vi "Configure Integer Display Dialog.vi"(7 "DisplayFilter":u8(ring)=7 items=["K_CHAN_R", "K_CHAN_W", "K_CHAN_RW", "K_CHAN_VOLT", "K_CHAN_FAULT", "K_ALL", "K_CUSTOM", "K_CHAN_R_VIS", "K_CHAN_W_VIS", "K_CHAN_RW_VIS", "K_CHAN_VOLT_VIS", "K_CHAN_FAULT_VIS"], 8 "error in (no error)":errorcluster, 9 "NIVS.System Definition Root":refnum<k24>, 11 "Data cluster in":T1={"Node Path"="", "NodePathArray"=[], "Integer"={"Label"="", "Digits of Precision"=0, "Integer Format"=enum."Scientific"}}) -> (0 "error out":errorcluster, 3 "Data cluster out":T1={"Node Path"="", "NodePathArray"=[], "Integer"={"Label"="", "Digits of Precision"=0, "Integer Format"=enum."Scientific"}})   [LabVIEW 2012]
doc: "Use this template to create a dialog box with event handling."
uses:
  NationalInstruments.VeriStand.SystemStorageUI
  NationalInstruments.VeriStand.SystemStorage
  <vilib>/NI Veristand/UI Controls/Single Node Browser/NI_VS UI Single Node Browser.lvlib
panel:
  in  "Integer Format":u8(ring) items=["Decimal"=0, "Scientific"=8, "Engineering"=2, "Binary"=3, "Octal"=4, "Hexadecimal"=5]
  in  "Digits of Precision":u8
  in  "Cancel":bool
  in  "Ok":bool
  in  "Selected Channel":refnum<k24>(container)
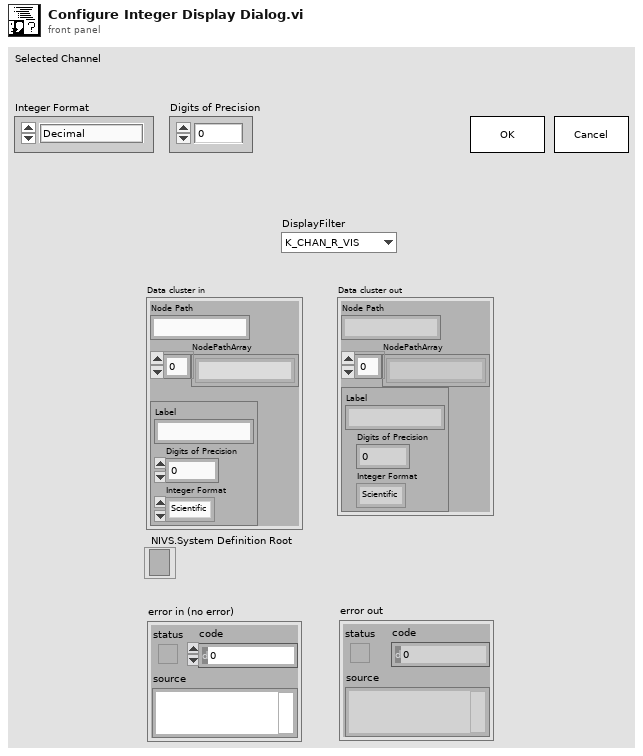
[diagram p1: front panel]
types:
  T1 = cluster{"Node Path":string, "NodePathArray":string[], "Integer":cluster{"Label":string, "Digits of Precision":u8, "Integer Format":enum8{"Decimal", "Scientific", "Engineering", "Binary", "Octal", "Hexadecimal", "Relative Time", "Time and Date", "SI"}}}
  T2 = enum8{"Decimal", "Scientific", "Engineering", "Binary", "Octal", "Hexadecimal", "Relative Time", "Time and Date", "SI"}
  T3 = typedef "NI_VS UI Single Node Browser.lvlib/Callback Type.ctl" = cluster{"Net Callbacks":refnum<k27>[], "Event":refnum<user-event>}
  T4 = typedef "NI_VS UI Single Node Browser.lvlib/Node Ref.ctl" = refnum<k24>
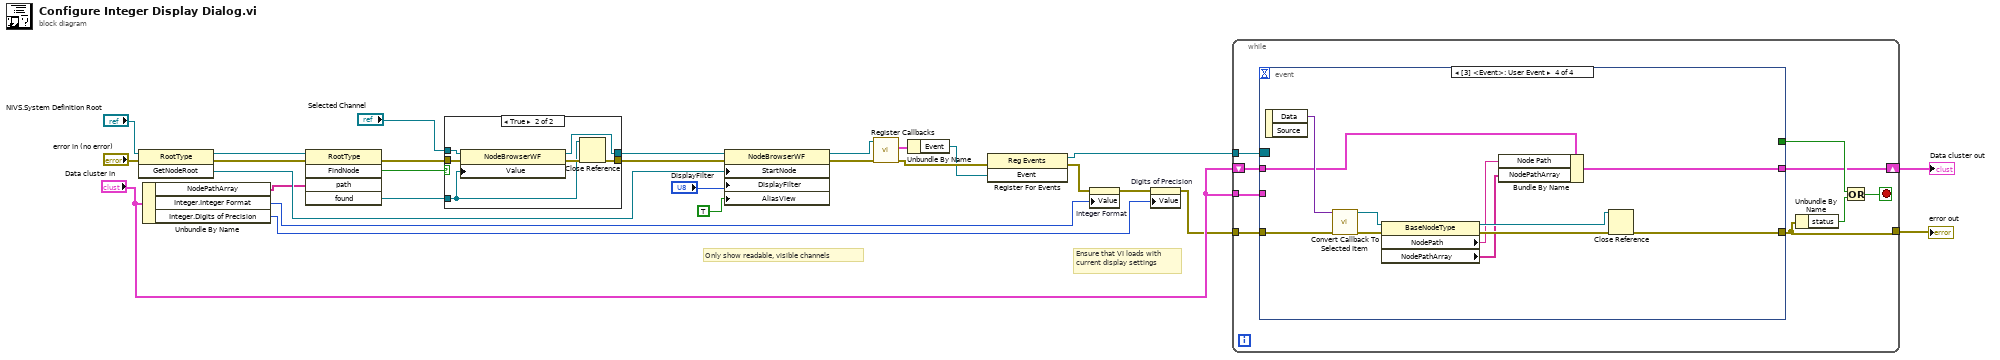
[diagram p0: block diagram]
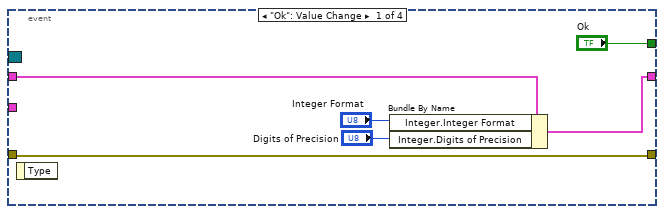
[diagram p3: hidden frame]
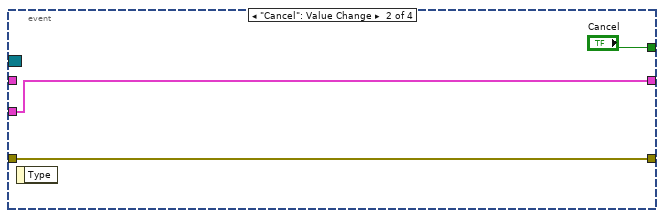
[diagram p4: hidden frame]
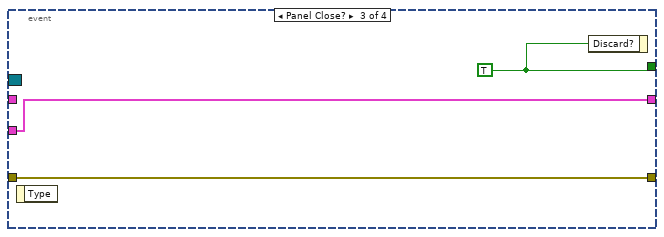
[diagram p5: hidden frame]
diagram:
  # "Ensure that VI loads with\ncurrent display settings"
  # "Only show readable, visible channels"
  n1 = invoke class="RootType" method="GetNodeRoot"(reference="NIVS.System Definition Root", error in="error in (no error)") -> (reference out=w22:refnum<k24>, error out=w23:errorcluster, "GetNodeRoot"=w21:refnum<k24>)  [unwired: 1 in]
  n2 = Unbundle By Name("Data cluster in") -> ("NodePathArray"=w8:string[], "Integer.Integer Format"=w2:T2, "Integer.Digits of Precision"=w1:u8)
  n3 = invoke class="RootType" method="FindNode"(reference=w22, error in=w23, "path"=w8) -> (error out=w14:errorcluster, "FindNode"=w12:bool, "found"=w15:refnum<k24>)  [unwired: 2 in, 2 out]
  n4 = case shown="True" w12 {
    tunnel: w15 -> [_ w31]
    tunnel: w14 -> [w30 w32]
    tunnel: [w30 w35] -> w13
    tunnel: "Selected Channel" -> [w29 w34]
    tunnel: [w29 w33] -> w11
    frame False {
    }
    frame True {
      n5 = property class="NodeBrowserWF"(reference=w34, error in=w32, "Value"=w31) -> (reference out=w33:refnum<k24>, error out=w36:errorcluster)
      n6 = Close Reference(reference=w31, error in (no error)=w36) -> (error out=w35:errorcluster)
    }
  }
  n7 = property class="NodeBrowserWF"(reference=w11, error in=w13, "StartNode"=w21, "DisplayFilter"="DisplayFilter", "AliasView"=TRUE) -> (reference out=w18:refnum<k24>, error out=w19:errorcluster)
  n8 = call <vilib>:"Register Callbacks.vi"("error in (no error)"=w19, "Single Node Browser"=w18) -> ("error out"=w27:errorcluster, "Callbacks"=w20:T3)  [unwired: 7 in, 1 out]
  n9 = Unbundle By Name(w20) -> ("Event"=w9:refnum<user-event>)
  n10 = register-events(error in=w27, w9) -> (reference out=w26:refnum<event-registration>, error out=w5:errorcluster)  [unwired: 1 in]
  n11 = property on="Integer Format" class="Ring (strict)"(error in=w5, "Value"=w2) -> (error out=w4:errorcluster)  [unwired: 1 in, 1 out]
  n12 = property on="Digits of Precision" class="DigNum (strict)"(error in=w4, "Value"=w1) -> (error out=w3:errorcluster)  [unwired: 1 in, 1 out]
  n13 = while {
    tunnel: [w43] -> w28
    tunnel: w3 -> [w44]
    tunnel: w26 -> [w41]
    shift-right: [w38] -> w6
    shift-left: "Data cluster in" -> [w40]
    tunnel: "Data cluster in" -> [w39]
    stop <- w37 stop-if-true
    n14 = event shown="[3] <Event>: User Event" {
      selector: w41 -> [_ _ _ _]
      dyn-events: _ -> [_ _ _ _]
      timeout: _ -> [_ _ _ _]
      tunnel: ["Ok" "Cancel" w55 _] -> w45
      tunnel: [w46 w53 w57 w66] -> w43
      tunnel: w44 -> [w46 w53 w57 w67]
      tunnel: w40 -> [w47 _ _ w60]
      tunnel: w39 -> [_ w52 w56 _]
      tunnel: [w48 w52 w56 w61] -> w38
      event "Ok": Value Change {
        n15 = event-data() -> ()  [unwired: 1 in, 1 out]
        n16 = Bundle By Name(cluster=w47, "Integer.Integer Format"="Integer Format", "Integer.Digits of Precision"="Digits of Precision") -> (w48:T1)
      }
      event "Cancel": Value Change {
        n17 = event-data() -> ()  [unwired: 1 in, 1 out]
      }
      event Panel Close? {
        w55 = TRUE ("Cancel")
        n18 = event-data() -> ()  [unwired: 1 in, 1 out]
        n19 = event-data("Discard?"=w55) -> ()  [unwired: 1 in, 1 out]
      }
      event User Event {
        n20 = event-data() -> ("Data"=w68:variant)  [unwired: 1 in, 1 out]
        n21 = call <vilib>:"Convert Callback To Selected Item.vi"("error in"=w67, "Data"=w68) -> ("error out"=w62:errorcluster, "Selected Item"=w65:T4)  [unwired: 8 in]
        n22 = property class="BaseNodeType"(reference=w65, error in=w62) -> (reference out=w64:T4, error out=w63:errorcluster, "NodePath"=w59:string, "NodePathArray"=w58:string[])
        n23 = Bundle By Name(cluster=w60, "Node Path"=w59, "NodePathArray"=w58) -> (w61:T1)
        n24 = Close Reference(reference=w64, error in (no error)=w63) -> (error out=w66:errorcluster)
      }
    }
    n25 = Unbundle By Name(w43) -> ("status"=w42:bool)
    n26 = Or(x=w45, y=w42) -> (x .or. y?=w37:bool)
  }
  "error out" <- w28
  "Data cluster out" <- w6
